vi "AddToPlaylist.vi"(6 "NewSong":string[](array[string]), 8 "error in":errorcluster, 9 "Playlist Clicked?":bool, 10 "Message Queues":T1, 11 "UI Refs":T2) -> (0 "error out":errorcluster)   [LabVIEW 2015]
uses:
  Controls & Type Defs/UI Data.ctl
  support/Message Queue/All Message Queues.ctl
  support/Message Queue/Message Cluster.ctl
  Controls & Type Defs/SongDetails.ctl
  support/Message Queue/Enqueue Message (Single).vi
  support/Message Queue/Message Queue.lvlib
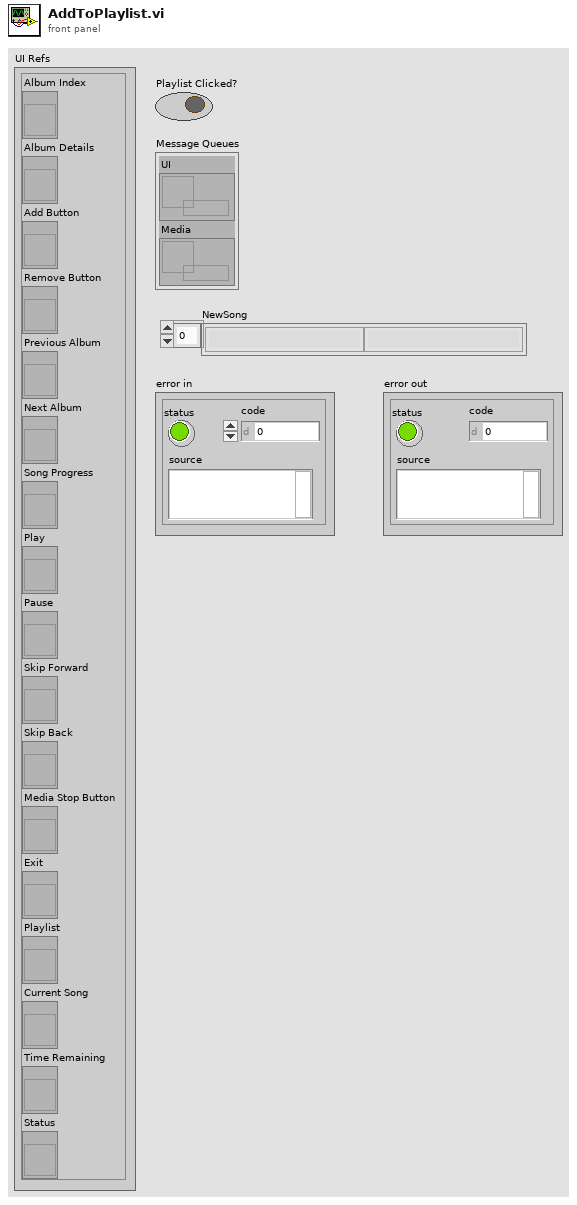
[diagram p1: front panel]
types:
  T1 = typedef "Message Queue.lvlib/All Message Queues.ctl" = cluster{"UI":refnum<queue>, "Media":refnum<queue>}
  T2 = typedef "UI Data.ctl" = cluster{"Album Index":refnum<vi>, "Album Details":refnum<vi>, "Add Button":refnum<vi>, "Remove Button":refnum<vi>, "Previous Album":refnum<vi>, "Next Album":refnum<vi>, "Song Progress":refnum<vi>, "Play":refnum<vi>, "Pause ":refnum<vi>, "Skip Forward":refnum<vi>, "Skip Back":refnum<vi>, "Media Stop Button":refnum<vi>, "Exit":refnum<vi>, "Playlist":refnum<vi>, "Current Song":refnum<vi>, "Time Remaining":refnum<vi>, "Status":refnum<vi>}
  T3 = typedef "AlbumDetails.ctl" = cluster{"Artist":string, "Album Name":string, "Songs":i32}
  T4 = typedef "SongDetails.ctl" = cluster{"Artist - Song Name":string, "Duration":string}
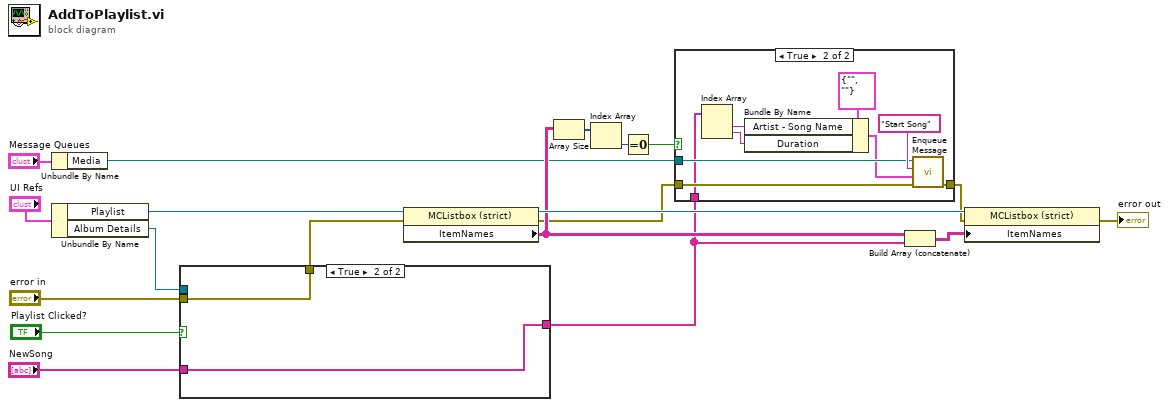
[diagram p0: block diagram]
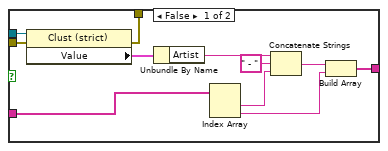
[diagram p3: hidden frame]
diagram:
  n1 = Unbundle By Name("Message Queues") -> ("Media"=w1:refnum<queue>)
  n2 = Unbundle By Name("UI Refs") -> ("Playlist"=w18:refnum<vi>, "Album Details"=w13:refnum<vi>)
  n3 = case shown="True" "Playlist Clicked?" {
    tunnel: "error in" -> [w30 w32]
    tunnel: w13 -> [w28 _]
    tunnel: [w27 w32] -> w12
    tunnel: "NewSong" -> [w26 w31]
    tunnel: [w20 w31] -> w3
    frame False {
      n4 = property class="Clust (strict)"(reference=w28, error in=w30) -> (error out=w27:errorcluster, "Value"=w29:T3)  [unwired: 1 out]
      n5 = Unbundle By Name(w29) -> ("Artist"=w25:string)
      n6 = Index Array(array=w26) -> (element #1=w24:string, element #2=w21:string)  [unwired: 2 in]
      n7 = Concatenate Strings(w25, " - " ("string"), w24) -> (w22:string)
      n8 = Build Array(w22, w21) -> (w20:string[])
    }
    frame True {
    }
  }
  n9 = property class="MCListbox (strict)"(reference=w18, error in=w12) -> (reference out=w17:refnum<vi>, error out=w5:errorcluster, "ItemNames"=w8:string[][])
  n10 = Array Size(array=w8) -> (size(s)=w7:i32[])
  n11 = Index Array(array=w7) -> (element=w6:i32)  [unwired: 1 in]
  n12 = Equal To 0?(x=w6) -> (x = 0?=w2:bool)
  n13 = case shown="True" w2 {
    tunnel: w5 -> [w33 w42]
    tunnel: [w33 w41] -> w4
    tunnel: w3 -> [_ w37]
    tunnel: w1 -> [_ w39]
    frame False {
    }
    frame True {
      n14 = Index Array(array=w37) -> (element #1=w36:string, element #2=w35:string)  [unwired: 2 in]
      n15 = Bundle By Name(cluster=T4 {"Artist - Song Name"="", "Duration"=""} ("Song Details"), "Artist - Song Name"=w36, "Duration"=w35) -> (w34:T4)
      n16 = call-poly "Enqueue Message.vi"("error in (no error)"=w42, "Message Data"=w34, "Message"="Start Song", "Message Queue"=w39) -> ("error out"=w41:errorcluster)  [unwired: 6 in, 1 out]
    }
  }
  n17 = Build Array (concatenate)(w8, w3) -> (w16:string[][])
  n18 = property class="MCListbox (strict)"(reference=w17, error in=w4, "ItemNames"=w16) -> (error out=→"error out":errorcluster)  [unwired: 1 out]
